vi "MovemotorMeng.vi"(8 "error in (no error)":errorcluster, 9 "lChanID":i32, 10 "Numeric":u32, 11 "Automation Refnum in":refnum<k7>) -> (0 "error out":errorcluster, 1 "Position":sgl, 3 "Automation Refnum out":refnum<k7>)   [LabVIEW 2014]
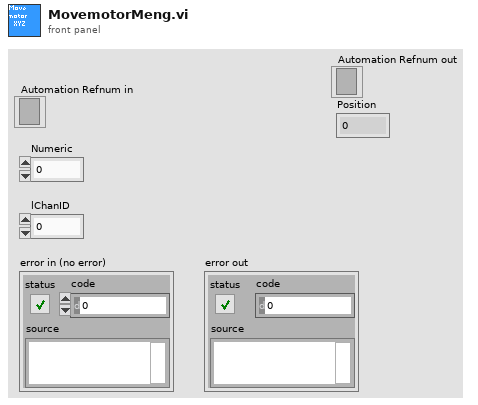
[diagram p1: front panel]
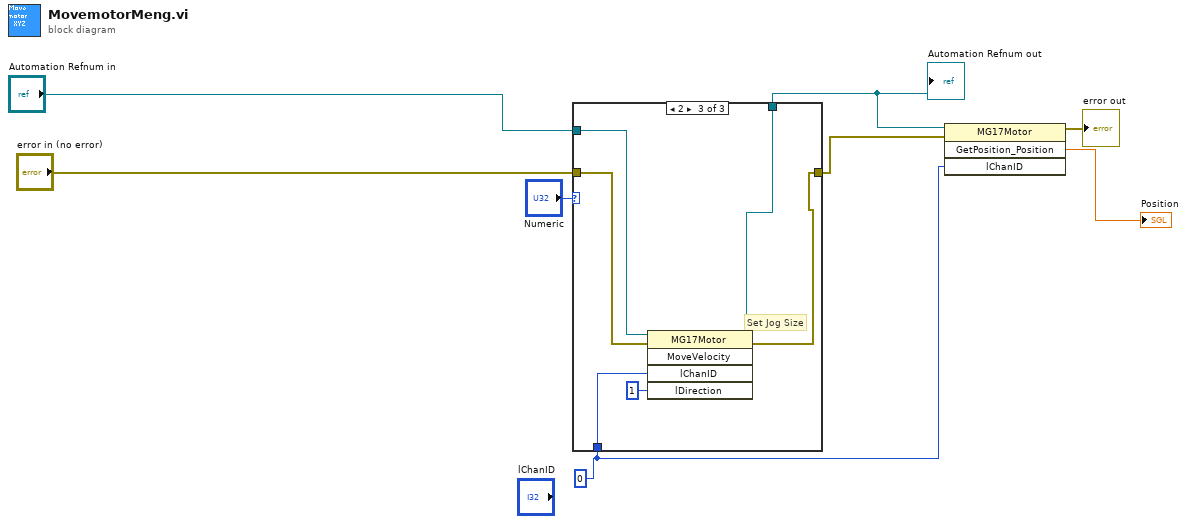
[diagram p0: block diagram]
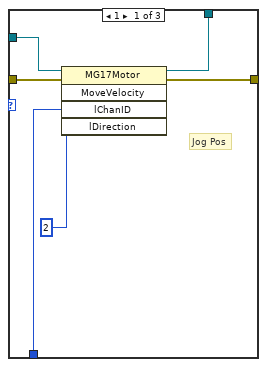
[diagram p2: hidden frame]
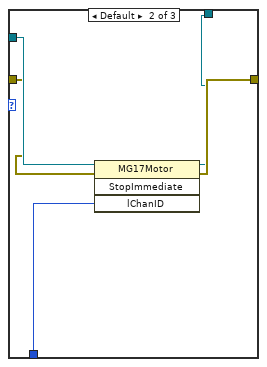
[diagram p3: hidden frame]
diagram:
  w1 = 0 ("lChanID")
  n1 = case shown="2" "Numeric" {
    tunnel: "Automation Refnum in" -> [w14 w19 w25]
    tunnel: w1 -> [w13 w16 w22]
    tunnel: [w12 w18 w23] -> w5
    tunnel: "error in (no error)" -> [w11 w17 w24]
    tunnel: [w9 w15 w20] -> w4
    frame 1 {
      # "Jog Pos"
      n2 = invoke class="MG17Motor" method="MoveVelocity"(reference=w14, error in=w11, "lChanID"=w13, "lDirection"=2) -> (reference out=w9:refnum<k7>, error out=w12:errorcluster)  [unwired: 1 in, 3 out]
    }
    frame Default {
      n3 = invoke class="MG17Motor" method="StopImmediate"(reference=w19, error in=w17, "lChanID"=w16) -> (reference out=w15:refnum<k7>, error out=w18:errorcluster)  [unwired: 1 in, 2 out]
    }
    frame 2 {
      # "Set Jog Size"
      n4 = invoke class="MG17Motor" method="MoveVelocity"(reference=w25, error in=w24, "lChanID"=w22, "lDirection"=1) -> (reference out=w20:refnum<k7>, error out=w23:errorcluster)  [unwired: 1 in, 3 out]
    }
  }
  "Automation Refnum out" <- w4
  n5 = invoke class="MG17Motor" method="GetPosition_Position"(reference=w4, error in=w5, "lChanID"=w1) -> (error out=→"error out":errorcluster, "GetPosition_Position"=→"Position":sgl)  [unwired: 1 in, 2 out]
